vi "Generate Archive Filepath.vi"(8 "error in (no error)":errorcluster) -> (0 "error out":errorcluster, 2 "Filepath":path, 3 "File Reference":refnum<file>)   [LabVIEW 2021]
uses:
  Type Definitions/Data Frame.ctl
  Type Definitions/Data Frame Header.ctl
  Type Definitions/Payload Class.ctl
  Type Definitions/Device.ctl
  Type Definitions/System Time.ctl
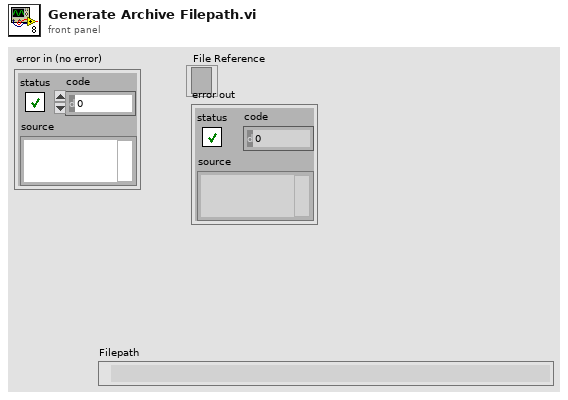
[diagram p1: front panel]
types:
  T1 = typedef "System Time.ctl" = cluster{"System Clock":timestamp, "GPS Clock":timestamp, "Nanosecond Counter":i64, "GPS Status":enum8{"Initializing", "Normal", "Unable to get fix"}, "GPS Antenna Status":enum8{"Unknown", "Normal", "Absent", "Overcurrent"}, "GPS Satelites Available":u8, "GPS Time (ns)":u64, "GPS UTC Offset":i8, "GPS Time Offset":i32, "UTC Offset Valid":bool, "GPS Time Lock":bool}
  T2 = typedef "Data Frame.ctl" = cluster{"Frame Header":T3, "Payload":string, "CRC":u32}
  T3 = typedef "Data Frame Header.ctl" = cluster{"Sync":u32, "Time":dbl, "Nanosecond Counter":i64, "Payload Class":T4, "Payload ID":u16, "Counter":i32, "Options":u32, "Source":T5, "Destination":T5}
  T4 = typedef "Payload Class.ctl" = enum16{"System State", "Parameters", "Metadata", "Software Monitor", "Data", "Commands"}
  T5 = typedef "Device.ctl" = enum32{"None", "Exec", "Aux1", "Aux2", "Aux3"}
  T6 = typedef "Disk State.ctl" = cluster{"File System Name":string, "Total":sgl, "Available":sgl, "Used":sgl, "Path":string}
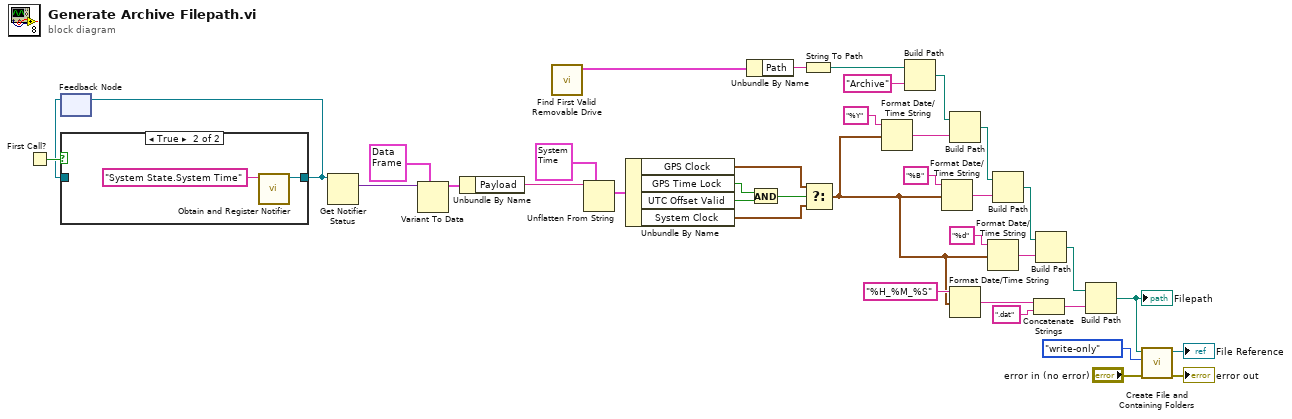
[diagram p0: block diagram]
diagram:
  n1 = First Call?() -> (First Call?: T/F=w15:bool)
  n2 = feedback #1() -> (w14:refnum<notifier>)  [unwired: 1 in]
  n3 = case shown="True" w15 {
    tunnel: [w39 w40] -> w13
    tunnel: w14 -> [w39 _]
    frame False {
    }
    frame True {
      n4 = call "Obtain and Register Notifier.vi"("name (unnamed)"="System State.System Time") -> ("notifier out"=w40:refnum<notifier>)  [unwired: 8 in, 2 out]
    }
  }
  n5 = feedback-in #1(w13) -> ()
  n6 = Get Notifier Status(notifier=w13) -> (current notification=w12:variant)  [unwired: 1 in, 4 out]
  n7 = Variant To Data(type=T2 {"Frame Header"={"Sync"=0, "Time"=0.0, "Nanosecond Counter"=0, "Payload Class"=enum."System State", "Payload ID"=0, "Counter"=0, "Options"=0, "Source"=enum."None", "Destination"=enum."None"}, "Payload"="", "CRC"=0} ("Frame"), Variant=w12) -> (data=w10:T2)  [unwired: 1 in, 1 out]
  n8 = Unbundle By Name(w10) -> ("Payload"=w9:string)
  n9 = call "Find First Valid Removable Drive.vi"() -> ("Disk State"=w16:T6)  [unwired: 11 in]
  n10 = Unflatten From String(type=T1 {"System Clock"=timestamp(0 s since 1904-01-01), "GPS Clock"=timestamp(0 s since 1904-01-01), "Nanosecond Counter"=0, "GPS Status"=enum."Initializing", "GPS Antenna Status"=enum."Unknown", "GPS Satelites Available"=0, "GPS Time (ns)"=0, "GPS UTC Offset"=0, "GPS Time Offset"=0, "UTC Offset Valid"=FALSE, "GPS Time Lock"=FALSE} ("System Time"), binary string=w9) -> (value=w7:T1)  [unwired: 3 in, 2 out]
  n11 = Unbundle By Name(w7) -> ("GPS Clock"=w3:timestamp, "GPS Time Lock"=w6:bool, "UTC Offset Valid"=w5:bool, "System Clock"=w2:timestamp)
  n12 = Unbundle By Name(w16) -> ("Path"=w18:string)
  n13 = And(x=w6, y=w5) -> (x .and. y?=w4:bool)
  n14 = String To Path(string=w18) -> (path=w17:path)
  n15 = Select(t=w3, s=w4, f=w2) -> (s? t:f=w1:timestamp)
  n16 = Format Date/Time String(time format string (%c)="%Y", seconds (now)=w1) -> (date/time string=w23:string)  [unwired: 1 in]
  n17 = Build Path(base path=w17, name or relative path="Archive" ("Folder Name")) -> (appended path=w33:path)
  n18 = Format Date/Time String(time format string (%c)="%B", seconds (now)=w1) -> (date/time string=w22:string)  [unwired: 1 in]
  n19 = Build Path(base path=w33, name or relative path=w23) -> (appended path=w32:path)
  n20 = Format Date/Time String(time format string (%c)="%H_%M_%S", seconds (now)=w1) -> (date/time string=w20:string)  [unwired: 1 in]
  n21 = Format Date/Time String(time format string (%c)="%d", seconds (now)=w1) -> (date/time string=w21:string)  [unwired: 1 in]
  n22 = Build Path(base path=w32, name or relative path=w22) -> (appended path=w31:path)
  n23 = Concatenate Strings(w20, ".dat" ("string")) -> (w29:string)
  n24 = Build Path(base path=w31, name or relative path=w21) -> (appended path=w30:path)
  n25 = Build Path(base path=w30, name or relative path=w29) -> (appended path=w28:path)
  "Filepath" <- w28
  n26 = call <vilib>:"Create File and Containing Folders.vi"("error in (no error)"="error in (no error)", "access"=enum16{"read/write", "read-only", "write-only"}."write-only", "file path"=w28) -> ("error out"=→"error out":errorcluster, "refnum out"=→"File Reference":refnum<file>)  [unwired: 7 in]
